vi "ExposeParameterListFromNameAndVariant.vi"(10 "Value Reference In":refnum<data-value>, 11 "Name (empty)":string) -> (0 "Value Reference Out":refnum<data-value>, 1 "Parmaeter Refs":refnum<data-value>[](array[refnum]), 3 "Parameter names":string[](array[string]))   [LabVIEW 2017]
uses:
  Mapper/ExposeObjectMapContainerTypeEnum.ctl
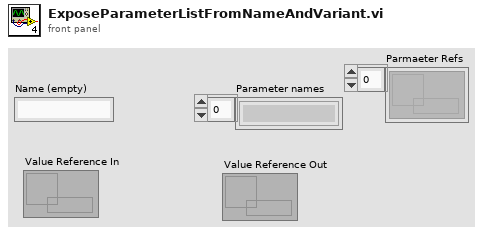
[diagram p1: front panel]
types:
  T1 = typedef "ExposeObjectMapContainerTypeEnum.ctl" = enum16{"Value", "Array", "Waveform", "NetContainer"}
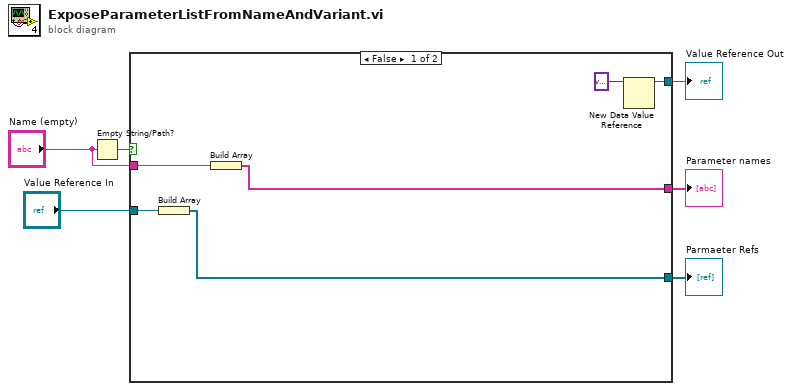
[diagram p0: block diagram]
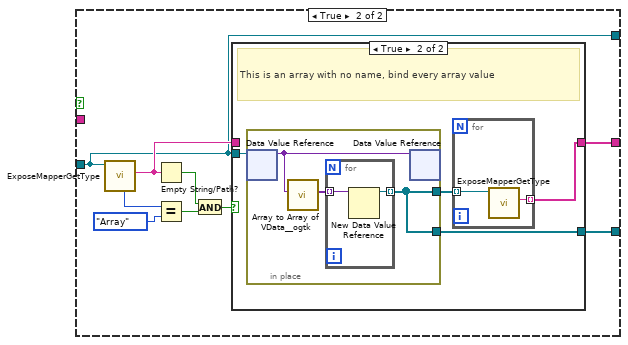
[diagram p2: hidden frame]
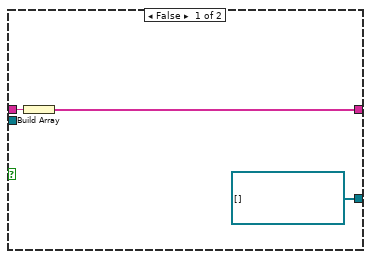
[diagram p3: hidden frame]
diagram:
  n1 = Empty String/Path?(string/path="Name (empty)") -> (empty?=w4:bool)
  n2 = case shown="False" w4 {
    tunnel: [w10 w14] -> w3
    tunnel: "Name (empty)" -> [w12 _]
    tunnel: [w11 w16] -> w6
    tunnel: "Value Reference In" -> [w9 w13]
    tunnel: [w7 w13] -> w1
    frame False {
      n3 = Build Array(w9) -> (w10:refnum<data-value>[])
      n4 = Build Array(w12) -> (w11:string[])
      n5 = New Data Value Reference(data value=variant) -> (data value reference=w7:refnum<data-value>)  [unwired: 1 in, 1 out]
    }
    frame True {
      n6 = call "ExposeMapperGetType.vi"("Data Val Ref in"=w13) -> ("Name"=w15:string, "Container Type (Labview Value type)"=w21:T1)  [unwired: 5 in, 4 out]
      n7 = Empty String/Path?(string/path=w15) -> (empty?=w19:bool)
      n8 = Equal?(x=w21, y=ExposeObjectMapContainerTypeEnum."Array") -> (x = y?=w18:bool)
      n9 = And(x=w19, y=w18) -> (x .and. y?=w17:bool)
      n10 = case shown="True" w17 {
        tunnel: w13 -> [_ w26]
        tunnel: [w23 w28] -> w16
        tunnel: w15 -> [w24 _]
        tunnel: [refnum<data-value>[] [] w27] -> w14
        frame False {
          n11 = Build Array(w24) -> (w23:string[])
        }
        frame True {
          # "This is an array with no name, bind every array value"
          n12 = in-place {
            in-place-border: [w29] -> w25
            in-place-border: [w29] -> w27
            n13 = in-place-dvr #1(w26) -> (w31:variant)  [unwired: 1 out]
            n14 = call <userlib>:"Array to Array of VData__ogtk.vi"("MultiD Array"=w31) -> ("1D Array of Variants"=w30:variant[])  [unwired: 9 in, 1 out]
            n15 = for {
              tunnel: w30 -> [w33] mode=indexing
              tunnel: [w32] -> w29 mode=indexing
              n16 = New Data Value Reference(data value=w33) -> (data value reference=w32:refnum<data-value>)  [unwired: 1 in, 1 out]
            }
            n17 = in-place-dvr #1(w31) -> ()  [unwired: 2 out]
          }
          n18 = for {
            tunnel: [w35] -> w28 mode=indexing
            tunnel: w25 -> [w34] mode=indexing
            n19 = call "ExposeMapperGetType.vi"("Data Val Ref in"=w34) -> ("Name"=w35:string)  [unwired: 5 in, 5 out]
          }
        }
      }
    }
  }
  "Parameter names" <- w6
  "Value Reference Out" <- w1
  "Parmaeter Refs" <- w3
